vi "Update.vi"(9 "Column":i32, 10 "Row":i32, 11 "64 in":refnum<class "64.lvclass">) -> (3 "64 out":refnum<class "64.lvclass">)   [LabVIEW 2015, in "64.lvclass"]
uses:
  64.lvclass
  64 Type.ctl
  Common/Position.ctl
  64.lvclass/64.ctl
  SubVIs/Read-Only Globals.vi
  SubVIs/Globals (private).vi
  Square/Square.lvclass
  Common/Common.lvlib
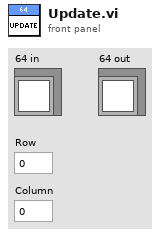
[diagram p1: front panel]
types:
  T1 = typedef "64.lvclass/64 Type.ctl" = enum16{"Starter", "Expander"}
  T2 = typedef "Common.lvlib/Position.ctl" = cluster{"Column":i32, "Row":i32}
  T3 = typedef "Common.lvlib/Map DVR.ctl" = refnum<data-value>
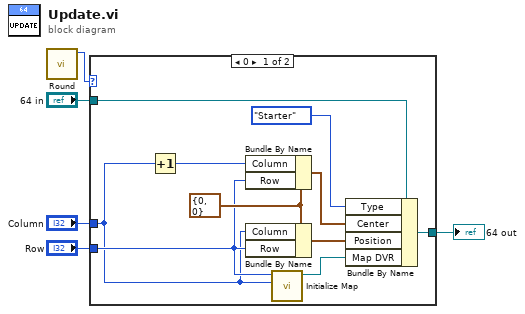
[diagram p0: block diagram]
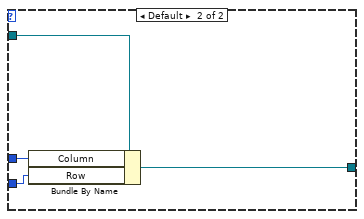
[diagram p2: hidden frame]
diagram:
  n1 = call "Round.vi"() -> ("Round"=w3:i32)  [unwired: 11 in]
  n2 = case shown="0" w3 {
    tunnel: "64 in" -> [w15 w19]
    tunnel: [w14 w18] -> w4
    tunnel: "Row" -> [w7 w16]
    tunnel: "Column" -> [w6 w17]
    frame 0 {
      w9 = T2 {"Column"=0, "Row"=0} ("Center")
      n3 = Increment(x=w6) -> (x+1=w12:i32)
      n4 = Bundle By Name(cluster=w9, "Column"=w12, "Row"=w7) -> (w11:T2)
      n5 = Bundle By Name(cluster=w9, "Column"=w6, "Row"=w7) -> (w10:T2)
      n6 = call "Initialize Map.vi"("Column"=w6, "Row"=w7) -> ("Map DVR"=w8:T3)  [unwired: 9 in]
      n7 = Bundle By Name(cluster=w15, "Type"=64_Type."Starter", "Center"=w11, "Position"=w10, "Map DVR"=w8) -> (w14:refnum<class "64.lvclass">)
    }
    frame Default {
      n8 = Bundle By Name(cluster=w19, "Column"=w17, "Row"=w16) -> (w18:refnum<class "64.lvclass">)
    }
  }
  "64 out" <- w4
